vi "Destroy Request Events.vi"(8 "error in":errorcluster) -> (0 "error out":errorcluster)   [LabVIEW 2025, in "USB IO.lvlib"]
doc: "Destroy the requests user events, even if there is an incoming error.\n\n<b>NOTE</b>: The contents of this VI are automatically generated and modified by the <b>Tools > DQMH Consortium > DQMH</b> utilities. Consider using those utilities instead of making your own modifications to this VI.\n_____\nBased on DQMH Dev Tools: Project Template 7.1.2.1547."
uses:
  USB IO.lvlib
panel:
  # "NOTE: The contents of this VI are automatically generated and modified by the Tools > DQMH Consortium > DQMH utilities. Consider using those utilities instead of making your own modifications to this VI."
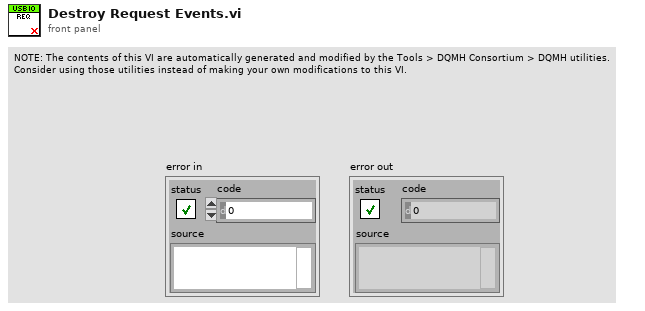
[diagram p1: front panel]
types:
  T1 = typedef "USB IO.lvlib/Request Events--cluster.ctl" = cluster{"Stop Module":refnum<user-event>, "Show Panel":refnum<user-event>, "Hide Panel":refnum<user-event>, "Show Diagram":refnum<user-event>, "Get Module Execution Status":refnum<user-event>, "Display Lines":refnum<user-event>, "select child":refnum<user-event>, "read config":refnum<user-event>, "init":refnum<user-event>, "init device":refnum<user-event>, "stop device":refnum<user-event>, "analog read":refnum<user-event>, "digital write":refnum<user-event>, "reconnect":refnum<user-event>}
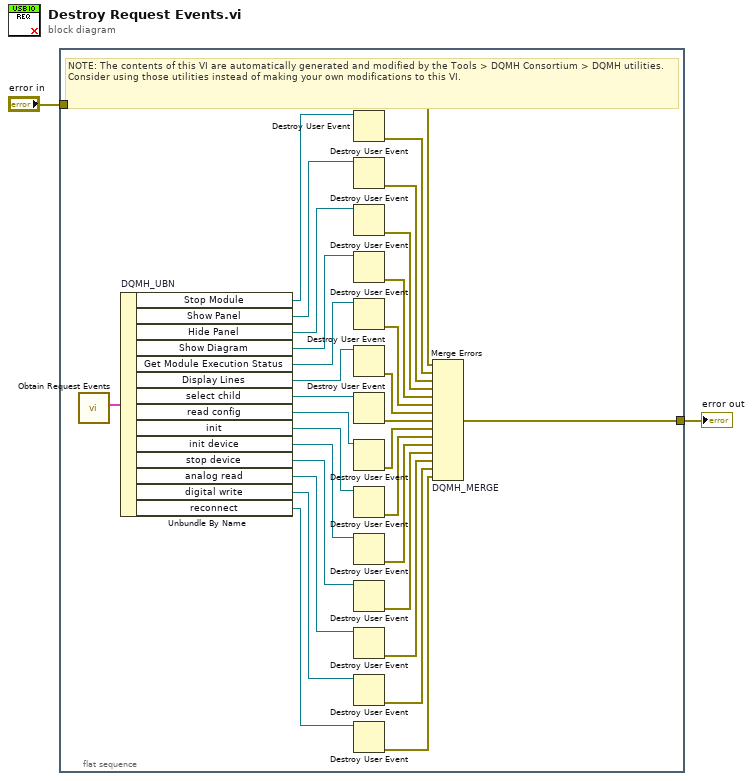
[diagram p0: block diagram]
diagram:
  n1 = flat-sequence {
    tunnel: [w32] -> w2
    tunnel: "error in" -> [w25]
    frame #0 {
      # "NOTE: The contents of this VI are automatically generated and modified by the Tools > DQMH Consortium > DQMH utilities. Consider using those utilities instead of making your own modifications to this VI."
      n2 = call "Obtain Request Events.vi"() -> ("USB IO Request Events"=w31:T1)  [unwired: 10 in, 1 out]
      n3 = Unbundle By Name "DQMH_UBN"(w31) -> ("Stop Module"=w30:refnum<user-event>, "Show Panel"=w27:refnum<user-event>, "Hide Panel"=w26:refnum<user-event>, "Show Diagram"=w23:refnum<user-event>, "Get Module Execution Status"=w21:refnum<user-event>, "Display Lines"=w19:refnum<user-event>, "select child"=w17:refnum<user-event>, "read config"=w15:refnum<user-event>, "init"=w13:refnum<user-event>, "init device"=w11:refnum<user-event>, "stop device"=w9:refnum<user-event>, "analog read"=w7:refnum<user-event>, "digital write"=w5:refnum<user-event>, "reconnect"=w3:refnum<user-event>)
      n4 = Destroy User Event(user event=w30) -> (error out=w33:errorcluster)  [unwired: 1 in]
      n5 = Destroy User Event(user event=w27) -> (error out=w29:errorcluster)  [unwired: 1 in]
      n6 = Destroy User Event(user event=w26) -> (error out=w28:errorcluster)  [unwired: 1 in]
      n7 = Destroy User Event(user event=w23) -> (error out=w24:errorcluster)  [unwired: 1 in]
      n8 = Destroy User Event(user event=w21) -> (error out=w22:errorcluster)  [unwired: 1 in]
      n9 = Destroy User Event(user event=w19) -> (error out=w20:errorcluster)  [unwired: 1 in]
      n10 = Destroy User Event(user event=w17) -> (error out=w18:errorcluster)  [unwired: 1 in]
      n11 = Destroy User Event(user event=w15) -> (error out=w16:errorcluster)  [unwired: 1 in]
      n12 = Destroy User Event(user event=w13) -> (error out=w14:errorcluster)  [unwired: 1 in]
      n13 = Destroy User Event(user event=w11) -> (error out=w12:errorcluster)  [unwired: 1 in]
      n14 = Destroy User Event(user event=w9) -> (error out=w10:errorcluster)  [unwired: 1 in]
      n15 = Destroy User Event(user event=w7) -> (error out=w8:errorcluster)  [unwired: 1 in]
      n16 = Destroy User Event(user event=w5) -> (error out=w6:errorcluster)  [unwired: 1 in]
      n17 = Destroy User Event(user event=w3) -> (error out=w4:errorcluster)  [unwired: 1 in]
      n18 = Merge Errors "DQMH_MERGE"(w25, w33, w29, w28, w24, w22, w20, w18, w16, w14, w12, w10, w8, w6, w4) -> (w32:errorcluster)
    }
  }
  "error out" <- w2
